vi "Write Image.vi"(0 "Session In":T1, 1 "Folder":string, 2 "Temp Image Name":string, 3 "Camera Missing?":bool, 5 "Error In":errorcluster, 6 "Student ID":i32) -> (14 "Session Out":T1, 16 "Image Out":T2, 19 "Error Out":errorcluster)   [LabVIEW 2013]
uses:
  <vilib>/vision/Image Controls.llb/IMAQ Image.ctl
  <vilib>/userdefined/High Color/IMAQdx.ctl
  <vilib>/vision/driver/NI_Vision_Acquisition_Software.lvlib
panel:
  out "appended path":path
  out "File Path":path
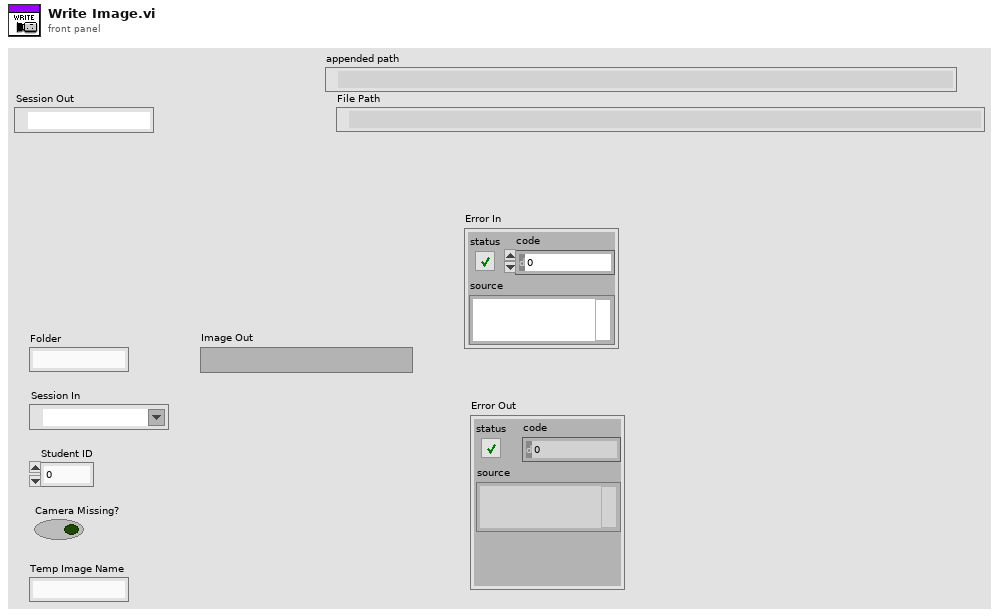
[diagram p1: front panel]
types:
  T1 = typedef "IMAQdx.ctl" = refnum<k21>
  T2 = typedef "IMAQ Image.ctl" = refnum<image>
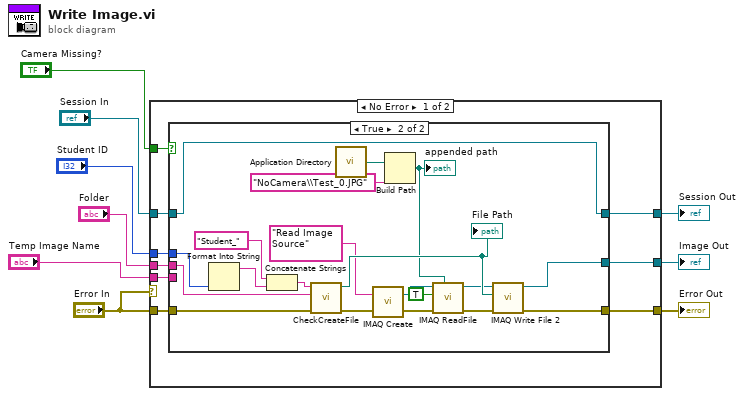
[diagram p0: block diagram]
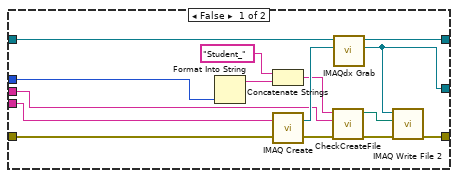
[diagram p2: hidden frame]
diagram:
  n1 = case shown="No Error" "Error In" {
    tunnel: "Temp Image Name" -> [w18 _]
    tunnel: "Folder" -> [w17 _]
    tunnel: "Student ID" -> [w16 _]
    tunnel: "Camera Missing?" -> [w15 _]
    tunnel: [w14 _] -> w5
    tunnel: "Session In" -> [w13 w54]
    tunnel: [w12 w54] -> w3
    tunnel: [w11 w55] -> w2
    tunnel: "Error In" -> [w10 w55]
    frame No Error {
      n2 = case shown="True" w15 {
        tunnel: w13 -> [w33 w48]
        tunnel: [w31 w41] -> w14
        tunnel: w16 -> [w26 w49]
        tunnel: w17 -> [w25 w45]
        tunnel: w18 -> [w24 _]
        tunnel: [w23 w48] -> w12
        tunnel: [w21 w38] -> w11
        tunnel: w10 -> [w20 w46]
        frame False {
          n3 = Format Into String(w26) -> (resulting string=w28:string)  [unwired: 3 in, 1 out]
          n4 = Concatenate Strings("Student_" ("string"), w28) -> (w27:string)
          n5 = call "IMAQ Create"("Image Name"=w24, "error in (no error)"=w20) -> ("New Image"=w32:T2, "error out"=w19:errorcluster)  [unwired: 2 in, 1 out]
          n6 = call "CheckCreateFile.vi"("Error In"=w19, "Folder"=w25, "Image Name"=w27) -> ("Error Out"=w22:errorcluster, "File Path"=w30:path)  [unwired: 7 in]
          n7 = call <vilib>:"IMAQdx Grab.vi"("Image In"=w32, "Session In"=w33) -> ("Image Out"=w31:T2, "Session Out"=w23:T1)  [unwired: 2 in, 6 out]
          n8 = call-poly "IMAQ Write File 2"("error in (no error)"=w22, "File Path"=w30, "Image"=w31) -> ("error out"=w21:errorcluster)  [unwired: 7 in, 1 out]
        }
        frame True {
          n9 = Format Into String(w49) -> (resulting string=w51:string)  [unwired: 3 in, 1 out]
          n10 = Concatenate Strings("Student_" ("string"), w51) -> (w50:string)
          n11 = call "CheckCreateFile.vi"("Error In"=w46, "Folder"=w45, "Image Name"=w50) -> ("Error Out"=w44:errorcluster, "File Path"=w53:path)  [unwired: 7 in]
          "File Path" <- w53
          n12 = call <vilib>:"Application Directory.vi"() -> ("Application Directory"=w37:path)
          n13 = call "IMAQ Create"("Image Name"="Read Image Source", "error in (no error)"=w44) -> ("New Image"=w40:T2, "error out"=w43:errorcluster)  [unwired: 3 in]
          n14 = Build Path(base path=w37, name or relative path="NoCamera\\Test_0.JPG") -> (appended path=w35:path)
          "appended path" <- w35
          n15 = call "IMAQ ReadFile"("File Path"=w35, "error in (no error)"=w43, "Load Color Palette? (No)"=TRUE, "Image"=w40) -> ("error out"=w42:errorcluster, "Image Out"=w39:T2)  [unwired: 3 in, 3 out]
          n16 = call-poly "IMAQ Write File 2"("error in (no error)"=w42, "File Path"=w53, "Image"=w39) -> ("error out"=w38:errorcluster, "Image Out (duplicate)"=w41:T2)  [unwired: 7 in]
        }
      }
    }
    frame Error {
      # "#Replace with Dummy \"Error\" Image"
    }
  }
  "Image Out" <- w5
  "Session Out" <- w3
  "Error Out" <- w2
